vi "Write Controller.vi"(8 "error in (no error)":errorcluster, 10 "Controller":refnum<class>, 11 "VIEW in":refnum<class "VIEW.lvclass">) -> (0 "error out":errorcluster, 3 "VIEW out":refnum<class "VIEW.lvclass">)   [LabVIEW 2013, in "VIEW.lvclass"]
uses:
  VIEW.lvclass
  VIEW.lvclass/VIEW.ctl
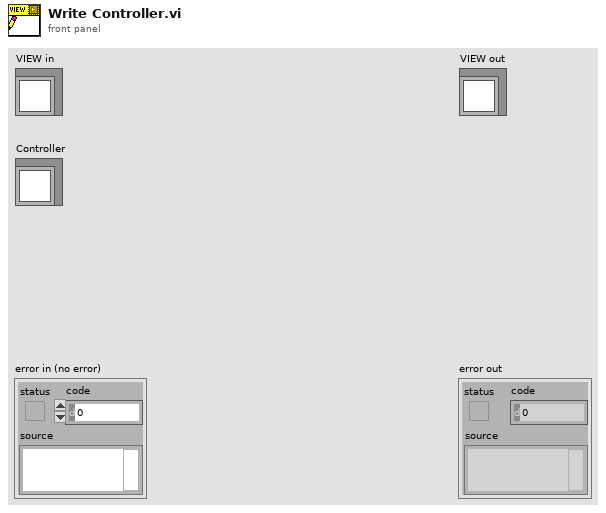
[diagram p1: front panel]
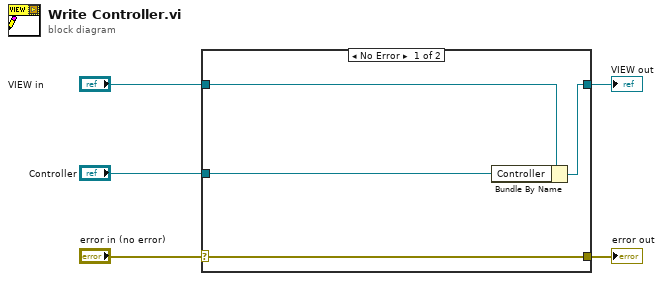
[diagram p0: block diagram]
diagram:
  n1 = case shown="No Error" "error in (no error)" {
    selector: "error in (no error)" -> [w9 w10]
    tunnel: [w9 w10] -> w4
    tunnel: [w7 w11] -> w2
    tunnel: "VIEW in" -> [w8 w11]
    tunnel: "Controller" -> [w6 _]
    frame No Error {
      n2 = Bundle By Name(cluster=w8, "Controller"=w6) -> (w7:refnum<class "VIEW.lvclass">)
    }
    frame Error {
    }
  }
  "error out" <- w4
  "VIEW out" <- w2
